vi "spi_single_master.vi"(7 "CPOL":bool=TRUE, 8 "SIG Port":refnum<k21>="Connector0/DIO0", 9 "CLK Port":refnum<k21>="Connector0/DIO1", 11 "Signal":bool=TRUE) -> (0 "SIG Port Out":refnum<k21>="Connector0/DIO0", 1 "CLK Port Out":refnum<k21>="Connector0/DIO1")   [LabVIEW 2013, in "kevLib2011.lvlib"]
uses:
  kevLib2011.lvlib
  <vilib>/rvi/eio/common/nirviEmuTemplateMethod_errors.vi
  <vilib>/eio/EIONode/EIONode.xnode
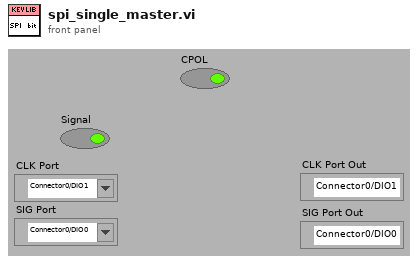
[diagram p1: front panel]
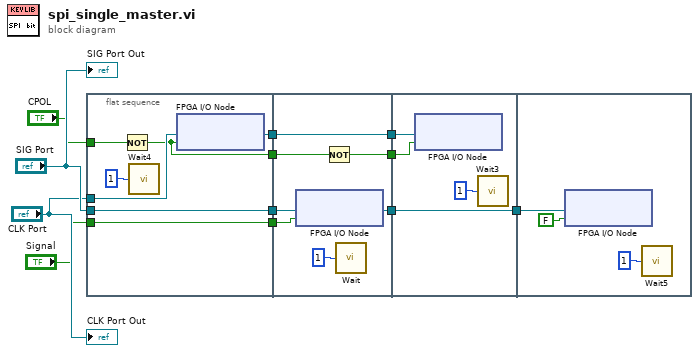
[diagram p0: block diagram]
diagram:
  n1 = flat-sequence {
    tunnel: "Signal" -> [w13]
    tunnel: "CPOL" -> [w17]
    tunnel: "CLK Port" -> [w18]
    tunnel: "SIG Port" -> [w14]
    tunnel: [w16] -> w7
    tunnel: [w15] -> w6
    tunnel: [w14] -> w4
    tunnel: [w13] -> w3
    tunnel: [w25] -> w8
    tunnel: w7 -> [w25]
    tunnel: w6 -> [w24]
    tunnel: [w23] -> w5
    tunnel: w4 -> [w22]
    tunnel: w3 -> [w21]
    tunnel: [w20] -> w1
    tunnel: w8 -> [w29]
    tunnel: w5 -> [w28]
    tunnel: [w27] -> w2
    tunnel: w1 -> [w27]
    tunnel: w2 -> [w31]
    frame #0 {
      n2 = Not(x=w17) -> (.not. x?=w15:bool)
      n3 = call "Wait4"("Count(uSec)"=u16 1) -> ()  [unwired: 1 out]
      n4 = xnode "FPGA I/O Node"("I/O Item"=w15, "FPGA I/O In"=w18) -> ("FPGA I/O Out"=w16:refnum<k21>)
    }
    frame #1 {
      n5 = xnode "FPGA I/O Node"("I/O Item"=w21, "FPGA I/O In"=w22) -> ("FPGA I/O Out"=w20:refnum<k21>)
      n6 = Not(x=w24) -> (.not. x?=w23:bool)
      n7 = call "Wait"("Count(uSec)"=u16 1) -> ()  [unwired: 1 out]
    }
    frame #2 {
      n8 = xnode "FPGA I/O Node"("I/O Item"=w28, "FPGA I/O In"=w29) -> ()  [unwired: 1 out]
      n9 = call "Wait3"("Count(uSec)"=u16 1) -> ()  [unwired: 1 out]
    }
    frame #3 {
      n10 = xnode "FPGA I/O Node"("I/O Item"=FALSE, "FPGA I/O In"=w31) -> ()  [unwired: 1 out]
      n11 = call "Wait5"("Count(uSec)"=u16 1) -> ()  [unwired: 1 out]
    }
  }
  "SIG Port Out" <- "SIG Port"
  "CLK Port Out" <- "CLK Port"
